vi "check_curvefit.vi"() -> ()   [LabVIEW 2013]
panel:
  in  "stop":bool
  out "fv":dbl format="%#_10g"
  in  "c":dbl step=0.01 format="%#_8g"
  in  "b":dbl step=0.001 format="%#_8g"
  in  "a":dbl step=0.01 format="%#_8g"
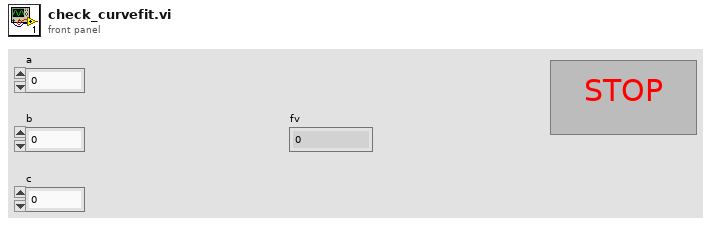
[diagram p1: front panel]
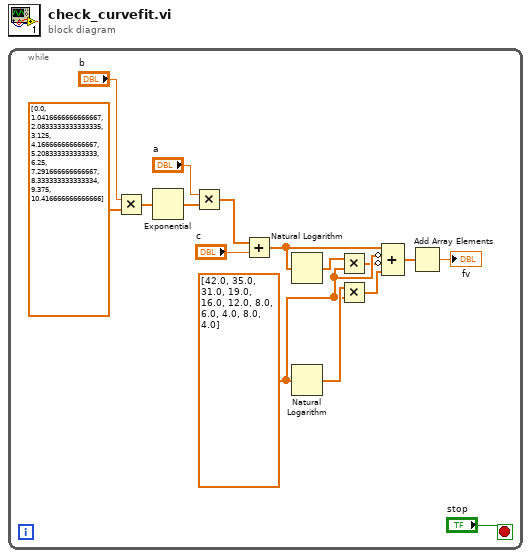
[diagram p0: block diagram]
diagram:
  n1 = while {
    stop <- "stop" stop-if-true
    w6 = dbl[] [42.0, 35.0, 31.0, 19.0, 16.0, 12.0, 8.0, 6.0, 4.0, 8.0, 4.0] ("x+y")
    n2 = Multiply(x="b", y=dbl[] [0.0, 1.0416666666666667, 2.0833333333333335, 3.125, 4.166666666666667, 5.208333333333333, 6.25, 7.291666666666667, 8.333333333333334, 9.375, 10.416666666666666] ("x+y")) -> (x*y=w12:dbl[])
    n3 = Exponential(1:w12) -> (0:w11:dbl[])
    n4 = Multiply(x="a", y=w11) -> (x*y=w14:dbl[])
    n5 = Add(x=w14, y="c") -> (x+y=w5:dbl[])
    n6 = Natural Logarithm(1:w5) -> (0:w8:dbl[])
    n7 = Natural Logarithm(1:w6) -> (0:w7:dbl[])
    n8 = Multiply(x=w8, y=w6) -> (x*y=w4:dbl[])
    n9 = Multiply(x=w7, y=w6) -> (x*y=w3:dbl[])
    n10 = Compound Arithmetic op=ADD(w5, invert w6, invert w4, w3) -> (w9:dbl[])
    n11 = Add Array Elements(numeric array=w9) -> (sum=→"fv":dbl)
  }
